vi "Teleop.vi"(10 "Match Info":T1={"Autonomous Elapsed Seconds"=0.0, "TeleOp Elapsed Seconds"=0.0, "Disabled Elapsed Seconds"=0.0, "Visited Autonomous"=FALSE, "Visited TeleOp"=FALSE, "Visited Disabled"=FALSE, "Autonomous Settings"={"Autonomous Style"=enum."Independent", "VI Refnum"=refnum}}, 11 "Call Context":T2) -> ()   [LabVIEW 2016]
doc: "This VI is called for each TeleOp packet received from the DS where the robot is not disabled. It is often used to read from the joysticks and update I/O or to update setpoints for timed control loops. It should complete and return within 20 milliseconds or it may miss DS packets."
uses:
  <vilib>/Rock Robotics/WPI/DriverStation/WPI_DriverStationDerivedRobotMode.ctl
  <vilib>/Rock Robotics/WPI/DriverStation/WPI_DriverStationMatch Info.ctl
  <vilib>/Rock Robotics/WPI/Solenoid/WPI_SolenoidValue.ctl
  <vilib>/Rock Robotics/Network Tables/NT Read Boolean.vi
  <vilib>/Rock Robotics/Network Tables/NT Read Number.vi
  <vilib>/Rock Robotics/WPI/Utilities/WPI_GetSetVariantRefNum.vi
  <vilib>/Rock Robotics/WPI/Joystick/WPI_JoystickArcadeMapping.vi
panel:
  in  "Boolean":bool=TRUE
  out "Sample Slider 0":dbl(slide) scale=0.0..5.0
  out "Sample Boolean 1":bool
  out "Sample Boolean 0":bool
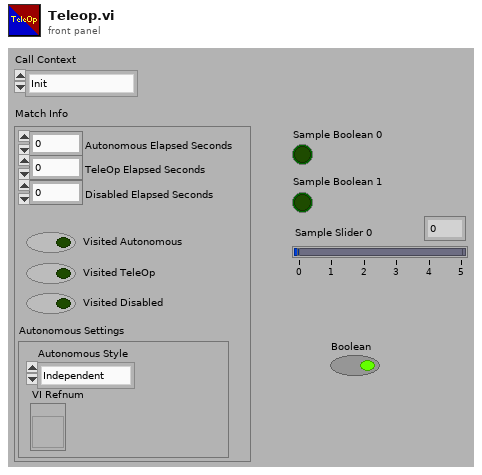
[diagram p1: front panel]
types:
  T1 = typedef "WPI_DriverStationMatch Info.ctl" = cluster{"Autonomous Elapsed Seconds":dbl, "TeleOp Elapsed Seconds":dbl, "Disabled Elapsed Seconds":dbl, "Visited Autonomous":bool, "Visited TeleOp":bool, "Visited Disabled":bool, "Autonomous Settings":cluster{"Autonomous Style":enum16{"Iterative", "Independent"}, "VI Refnum":refnum<vi>}}
  T2 = typedef "WPI_DriverStationDerivedRobotMode.ctl" = enum16{"Init", "Execute", "Stop"}
  T3 = typedef "WPI_JoystickDevRef.ctl" = cluster{"Device":T4}
  T4 = typedef "WPI_JoystickDeviceEnum.ctl" = enum16{"USB 0", "USB 1", "USB 2", "USB 3", "USB 4", "USB 5"}
  T5 = cluster{"Gyro":string, "Mtr 1":string, "Mtr 2":string}
  T6 = typedef "WPI_SolenoidValue.ctl" = enum16{"Off", "On", "Forward", "Reverse"}
  T7 = typedef "WPI_SolenoidDevRef.ctl" = cluster{"DevStatus":errorcluster, "Pneumatics Control Module":u8, "Forward Solenoid Channel":T8, "Reverse Solenoid Channel":T8}
  T8 = typedef "WPI_SolenoidChannel.ctl" = enum8{"Solenoid 0", "Solenoid 1", "Solenoid 2", "Solenoid 3", "Solenoid 4", "Solenoid 5", "Solenoid 6", "Solenoid 7", "Invalid"}
  T9 = typedef "WPI_MotorControlDeviceRef.ctl" = cluster{"DeviceStatus":errorcluster, "Type":T10, "PWM":cluster{"PWM Channel":T11, "DeadBand":T12}, "CAN":cluster{"Device Number":u8, "SetOutput VI Ref":variant, "GetOutput VI Ref":variant, "Enable VI Ref":variant, "Disable VI Ref":variant, "Data":variant}, "Invert":bool}
  T10 = typedef "WPI_MotorControlType.ctl" = enum16{"PWM", "CAN"}
  T11 = typedef "FPGA_DIOPWMChannel.ctl" = enum8{"PWM 0", "PWM 1", "PWM 2", "PWM 3", "PWM 4", "PWM 5", "PWM 6", "PWM 7", "PWM 8", "PWM 9", "PWM MXP 0", "PWM MXP 1", "PWM MXP 2", "PWM MXP 3", "PWM MXP 4", "PWM MXP 5", "PWM MXP 6", "PWM MXP 7", "PWM MXP 8", "PWM MXP 9", "Invalid"}
  T12 = typedef "WPI_PWMDeadband.ctl" = cluster{"Name":string, "maxPositivePwm":i32, "minPositivePwm":i32, "centerPwm":i32, "maxNegativePwm":i32, "minNegativePwm":i32, "angularRange":u16}
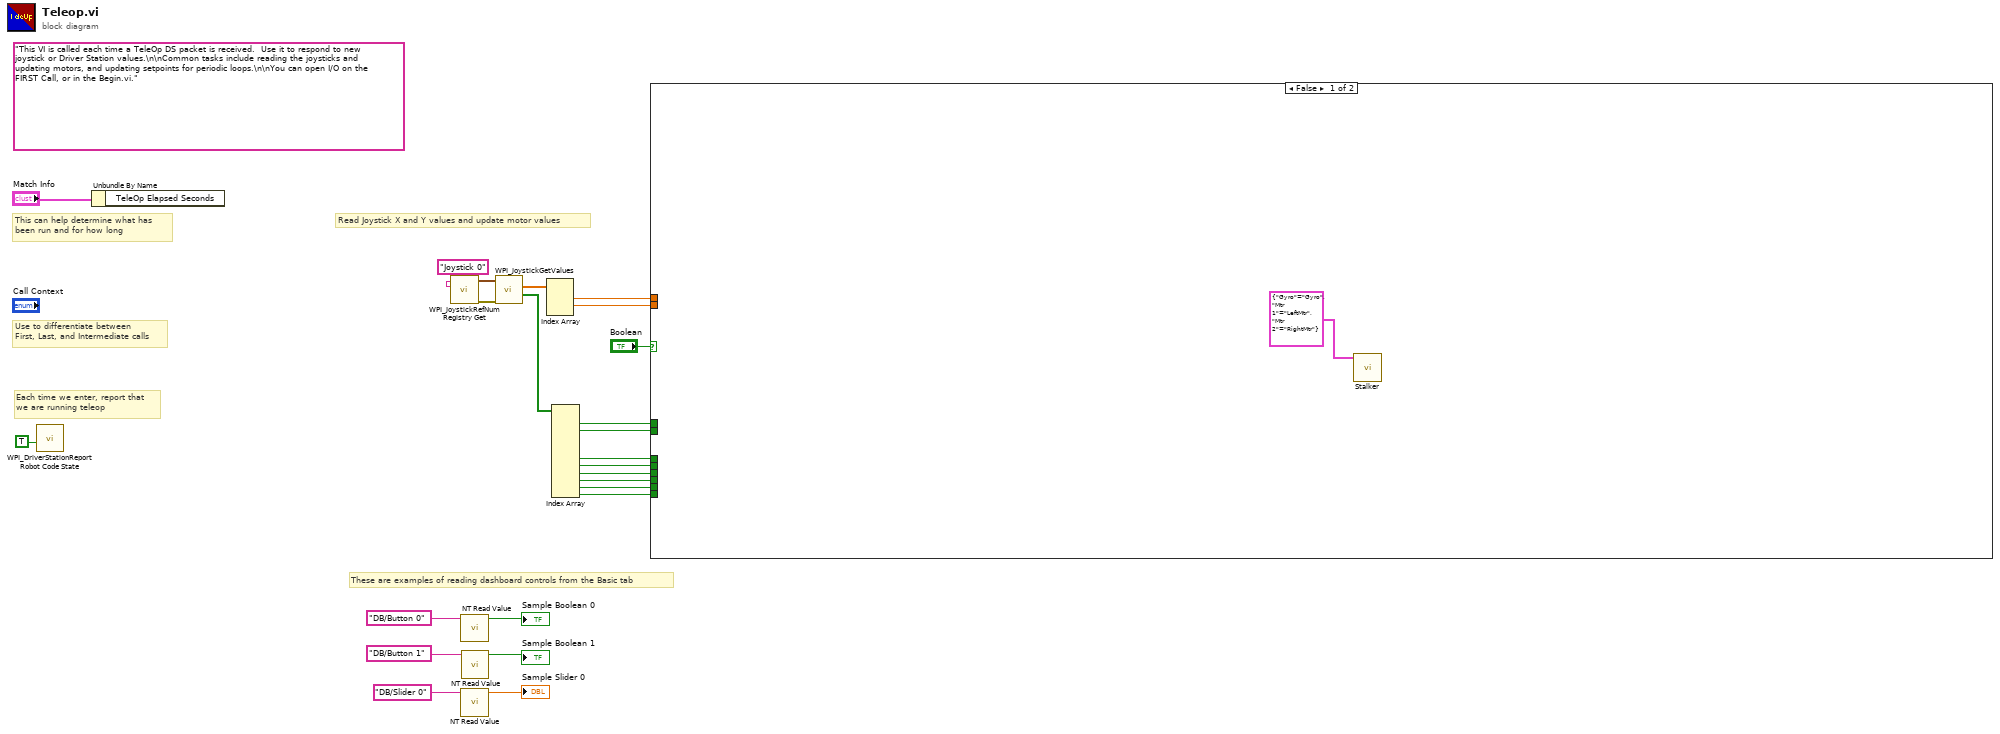
[diagram p0: block diagram]
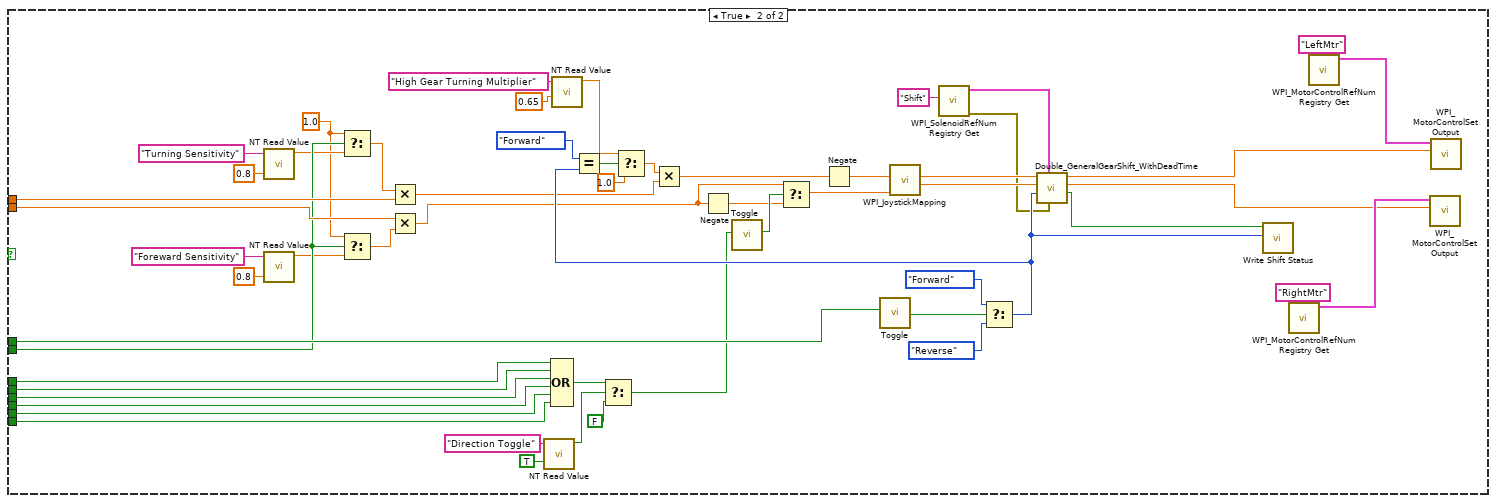
[diagram p2: hidden frame]
diagram:
  (unwired) "This VI is called each time a TeleOp DS packet is received.  Use it to respond to new joystick or Driver Station values.\n\nCommon tasks include reading the joysticks and updating motors, and updating setpoints for periodic loops.\n\nYou can open I/O on the FIRST Call, or in the Begin.vi."
  # "These are examples of reading dashboard controls from the Basic tab"
  # "Each time we enter, report that\nwe are running teleop"
  # "Use to differentiate between\nFirst, Last, and Intermediate calls"
  # "This can help determine what has\nbeen run and for how long"
  # "Read Joystick X and Y values and update motor values"
  n1 = call <vilib>:"WPI_DriverStationReport Robot Code State.vi"("TeleOp"=TRUE ("Autonomous")) -> ()  [unwired: 10 in, 1 out]
  n2 = Unbundle By Name("Match Info") -> ()  [unwired: 1 out]
  n3 = call <vilib>:"WPI_JoystickRefNum Registry Get.vi"("refnum name"="Joystick 0") -> ("error out"=w13:errorcluster, "JoystickDevRef"=w16:T3)  [unwired: 1 in, 8 out]
  n4 = call-poly <vilib>:"NT Read Value.vi"("Name"="DB/Button 0" ("refnum name")) -> ("Boolean"=→"Sample Boolean 0":bool)  [unwired: 9 in, 1 out]
  n5 = call-poly <vilib>:"NT Read Value.vi"("Name"="DB/Slider 0" ("refnum name")) -> ("Numeric"=→"Sample Slider 0":dbl)  [unwired: 9 in, 1 out]
  n6 = call-poly <vilib>:"NT Read Value.vi"("Name"="DB/Button 1" ("refnum name")) -> ("Boolean"=→"Sample Boolean 1":bool)  [unwired: 9 in, 1 out]
  n7 = call <vilib>:"WPI_JoystickGetValues.vi"("error in (no error)"=w13, "JoystickDevRef"=w16) -> ("Buttons"=w14:bool[], "Axes"=w15:dbl[])  [unwired: 5 in, 3 out]
  n8 = Index Array(array=w15) -> (element #1=w5:dbl, element #2=w4:dbl)  [unwired: 3 in, 1 out]
  n9 = Index Array(array=w14) -> (element #1=w6:bool, element #2=w3:bool, element #6=w12:bool, element #7=w11:bool, element #8=w10:bool, element #9=w9:bool, element #10=w7:bool, element #11=w8:bool)  [unwired: 11 in, 3 out]
  n10 = case shown="False" "Boolean" {
    tunnel: w12 -> [_ w80]
    tunnel: w11 -> [_ w79]
    tunnel: w10 -> [_ w78]
    tunnel: w9 -> [_ w77]
    tunnel: w8 -> [_ w76]
    tunnel: w7 -> [_ w75]
    tunnel: w6 -> [_ w68]
    tunnel: w5 -> [_ w65]
    tunnel: w4 -> [_ w64]
    tunnel: w3 -> [_ w63]
    frame False {
      n11 = call "Stalker.vi"("Refnum's In"=T5 {"Gyro"="Gyro", "Mtr 1"="LeftMtr", "Mtr 2"="RightMtr"}) -> ()  [unwired: 9 in, 2 out]
    }
    frame True {
      w29 = 1.0 ("t")
      n12 = call-poly <vilib>:"NT Read Value.vi"("Default Value"=0.8, "Name"="Turning Sensitivity") -> ("Numeric"=w31:dbl)  [unwired: 8 in, 1 out]
      n13 = call-poly <vilib>:"NT Read Value.vi"("Default Value"=0.8, "Name"="Foreward Sensitivity") -> ("Numeric"=w33:dbl)  [unwired: 8 in, 1 out]
      n14 = Select(t=w29, s=w63, f=w31) -> (s? t:f=w30:dbl)
      n15 = Select(t=w29, s=w63, f=w33) -> (s? t:f=w32:dbl)
      n16 = Multiply(x=w30, y=w65) -> (x*y=w34:dbl)
      n17 = Multiply(x=w64, y=w32) -> (x*y=w35:dbl)
      n18 = call-poly <vilib>:"NT Read Value.vi"("Default Value"=TRUE, "Name"="Direction Toggle") -> ("Boolean"=w46:bool)  [unwired: 8 in, 1 out]
      n19 = Compound Arithmetic op=OR(w80, w79, w78, w77, w75, w76) -> (w47:bool)
      n20 = call-poly <vilib>:"NT Read Value.vi"("Default Value"=0.65, "Name"="High Gear Turning Multiplier") -> ("Numeric"=w41:dbl)  [unwired: 8 in, 1 out]
      n21 = Select(t=w47, s=w46, f=FALSE) -> (s? t:f=w43:bool)
      n22 = Negate(x=w35) -> (-x=w61:dbl)
      n23 = call "Toggle.vi"("Input"=w43) -> ("Output"=w62:bool)  [unwired: 10 in]
      n24 = Select(t=w35, s=w62, f=w61) -> (s? t:f=w28:dbl)
      n25 = call "Toggle.vi"("Input"=w68) -> ("Output"=w58:bool)  [unwired: 10 in]
      n26 = call <vilib>:"WPI_SolenoidRefNum Registry Get.vi"("refnum name"="Shift") -> ("error out"=w53:errorcluster, "SolenoidDevRef"=w54:T7)  [unwired: 9 in]
      n27 = Select(t=WPI_SolenoidValue."Forward" ("Shift Value"), s=w58, f=WPI_SolenoidValue."Reverse" ("Shift Value")) -> (s? t:f=w66:T6)
      n28 = Equal?(x=WPI_SolenoidValue."Forward" ("Shift Value"), y=w66) -> (x = y?=w52:bool)
      n29 = Select(t=w41, s=w52, f=1.0) -> (s? t:f=w49:dbl)
      n30 = Multiply(x=w49, y=w34) -> (x*y=w27:dbl)
      n31 = Negate(x=w27) -> (-x=w26:dbl)
      n32 = call-poly <vilib>:"WPI_JoystickMapping.vi"("Y axis value"=w28, "X axis value"=w26) -> ("Right Motor Value"=w59:dbl, "Left Motor Value"=w60:dbl)  [unwired: 8 in]
      n33 = call "Double_GeneralGearShift_WithDeadTime.vi"("error In"=w53, "ShifterRef"=w54, "Shift Value"=w66, "Right"=w59, "Left"=w60) -> ("Shifting"=w67:bool, "Right Output"=w69:dbl, "Left Output"=w70:dbl)  [unwired: 3 in, 1 out]
      n34 = call "Write Shift Status.vi"("Gear"=w66, "Output"=w67) -> ()  [unwired: 9 in, 1 out]
      n35 = call <vilib>:"WPI_MotorControlRefNum Registry Get.vi"("refnum name"="RightMtr") -> ("MotorControlDevRef"=w73:T9)  [unwired: 9 in, 1 out]
      n36 = call <vilib>:"WPI_MotorControlRefNum Registry Get.vi"("refnum name"="LeftMtr") -> ("MotorControlDevRef"=w74:T9)  [unwired: 9 in, 1 out]
      n37 = call <vilib>:"WPI_MotorControlSetOutput.vi"("Output"=w69, "MotorControlDevRef"=w73) -> ()  [unwired: 7 in, 3 out]
      n38 = call <vilib>:"WPI_MotorControlSetOutput.vi"("Output"=w70, "MotorControlDevRef"=w74) -> ()  [unwired: 7 in, 3 out]
    }
  }
